vi "Discovery Listener.vi"(0 "stop notifier":refnum<notifier>, 5 "discoveryPort":u16=10001, 7 "Discovery Events":T1) -> (15 "error out":errorcluster)   [LabVIEW 2020, in "epl-network.lvlib"]
uses:
  epl-network.lvlib
  Discovery Events.ctl
  Discovered Host.ctl
  Public/Discovery/Typedefs/Server Beacon.ctl
  bf470879-c08b-4c96-b320-132c7bb87e46.vi
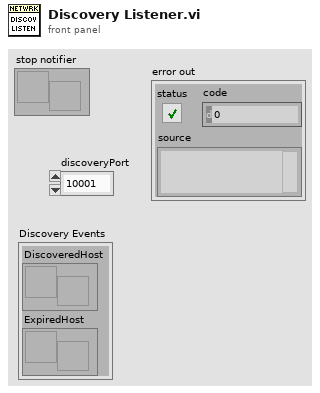
[diagram p1: front panel]
types:
  T1 = typedef "epl-network.lvlib/Discovery Events.ctl" = cluster{"DiscoveredHost":refnum<user-event>, "ExpiredHost":refnum<user-event>}
  T2 = typedef "epl-network.lvlib/Discovered Host.ctl" = cluster{"Beacon":T3, "Last Seen":timestamp}
  T3 = typedef "epl-network.lvlib/Server Beacon.ctl" = cluster{"name":string, "addr":string, "port":u16, "ver":u16}
  T4 = cluster{"DiscoveryBeacon":T3, "seconds since 1Jan1904":timestamp}
  T5 = typedef "epl-network.lvlib/Beacon Result.ctl" = enum16{"Ignored", "Updated", "Added"}
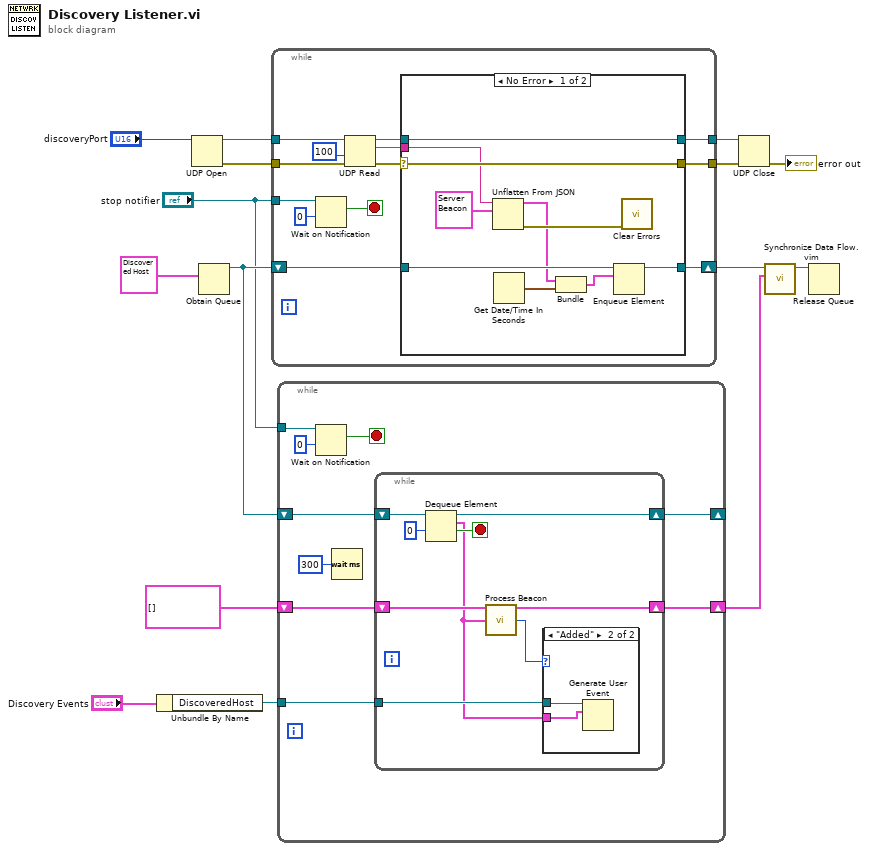
[diagram p0: block diagram]
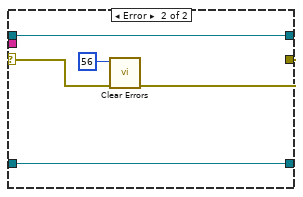
[diagram p3: hidden frame]
diagram:
  n1 = Unbundle By Name("Discovery Events") -> ("DiscoveredHost"=w5:refnum<user-event>)
  n2 = UDP Open(11:"discoveryPort") -> (port=w12:refnum<k16>, 0:w13:errorcluster)  [unwired: 4 in, 1 out]
  n3 = Obtain Queue(element data type=T2 {"Beacon"={"name"="", "addr"="", "port"=0, "ver"=10001}, "Last Seen"=timestamp(0 s since 1904-01-01)} ("DiscoveredHost")) -> (queue out=w9:refnum<queue>)  [unwired: 4 in, 2 out]
  n4 = while {
    tunnel: w12 -> [w28]
    tunnel: w13 -> [w27]
    tunnel: [w26] -> w14
    tunnel: [w25] -> w15
    tunnel: "stop notifier" -> [w20]
    shift-right: [w18] -> w4
    shift-left: w9 -> [w19]
    stop <- w17 stop-if-true
    n5 = Wait on Notification(notifier=w20, timeout in ms (-1)=0) -> (notification=w17:bool)  [unwired: 2 in, 3 out]
    n6 = UDP Read(connection ID=w28, timeout ms (25000)=100, 8:w27) -> (data out=w22:string, error out=w23:errorcluster, 3:w21:refnum<k16>)  [unwired: 3 out]
    n7 = case shown="No Error" w23 {
      selector: w23 -> [w37 w43]
      tunnel: [w37 w41] -> w26
      tunnel: w22 -> [w36 _]
      tunnel: w21 -> [w38 w40]
      tunnel: [w38 w40] -> w25
      tunnel: w19 -> [w33 w39]
      tunnel: [w32 w39] -> w18
      frame No Error {
        n8 = Unflatten From JSON(JSON string=w36, type and defaults=T3 {"name"="", "addr"="192.168.1.98", "port"=57469, "ver"=10001} ("DiscoveryBeacon")) -> (value=w31:T3, error out=w34:errorcluster)  [unwired: 5 in]
        n9 = Get Date/Time In Seconds() -> (seconds since 1Jan1904=w30:timestamp)
        n10 = Bundle("DiscoveryBeacon"=w31, "seconds since 1Jan1904"=w30) -> (w29:T4)  [unwired: 1 in]
        n11 = Enqueue Element(queue=w33, element=w29) -> (queue out=w32:refnum<queue>)  [unwired: 2 in, 2 out]
        n12 = call <vilib>:"Clear Errors.vi"("error in (no error)"=w34) -> ()  [unwired: 5 in, 2 out]
      }
      frame Error {
        n13 = call <vilib>:"Clear Errors.vi"("error in (no error)"=w43, "specific error code to clear (0: all)"=56) -> ("error out"=w41:errorcluster)  [unwired: 4 in, 1 out]
      }
    }
  }
  n14 = while {
    shift-right: [w50] -> _
    shift-left: w9 -> [w52]
    shift-right: [w48] -> w2
    shift-left: T2[] [] ("Array") -> [w51]
    tunnel: w5 -> [w49]
    tunnel: "stop notifier" -> [w45]
    stop <- w44 stop-if-true
    n15 = Wait on Notification(notifier=w45, timeout in ms (-1)=0) -> (notification=w44:bool)  [unwired: 2 in, 3 out]
    n16 = Wait (ms)(milliseconds to wait=u32 300) -> ()  [unwired: 1 out]
    n17 = while {
      shift-right: [w59] -> w50
      shift-left: w52 -> [w61]
      shift-right: [w56] -> w48
      shift-left: w51 -> [w57]
      tunnel: w49 -> [w54]
      stop <- w58 stop-if-true
      n18 = Dequeue Element(queue=w61, timeout in ms (-1)=0) -> (queue out=w59:refnum<queue>, element=w53:T2, timed out?=w58:bool)  [unwired: 1 in, 1 out]
      n19 = call "Process Beacon.vi"("Known Hosts in"=w57, "DiscoveredHost"=w53) -> ("Known Hosts out"=w56:T2[], "Beacon Result"=w55:T5)  [unwired: 12 in]
      n20 = case shown="\"Added\"" w55 {
        tunnel: w54 -> [_ w63]
        tunnel: w53 -> [_ w62]
        frame "Ignored", Default {
        }
        frame "Added" {
          n21 = Generate User Event(user event=w63, event data cluster=w62) -> ()  [unwired: 2 in, 2 out]
        }
      }
    }
  }
  n22 = UDP Close(connection ID=w15, 8:w14) -> (error out=→"error out":errorcluster)  [unwired: 1 out]
  n23 = call "Synchronize Data Flow.vim"("input 2"=w2, "input 1"=w4) -> ("output 1"=w3:refnum<queue>)  [unwired: 2 in, 3 out]
  n24 = Release Queue(queue=w3) -> ()  [unwired: 2 in, 3 out]
